vi "Format Metadata.vi"(0 "Tone Cloud in":refnum<class "Tone Cloud.lvclass">, 7 "Prefix":string, 11 "error in (no error)":errorcluster) -> (4 "Tone Cloud out":refnum<class "Tone Cloud.lvclass">, 8 "String":string, 15 "error out":errorcluster)   [LabVIEW 2020, in "Tone Cloud.lvclass"]
uses:
  Tone Cloud.lvclass
  Tone Cloud.lvclass/Tone Cloud.ctl
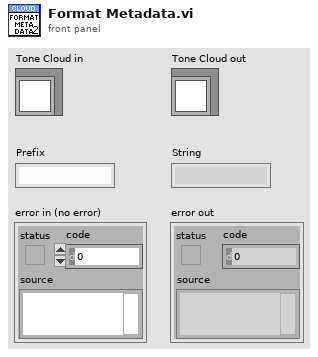
[diagram p1: front panel]
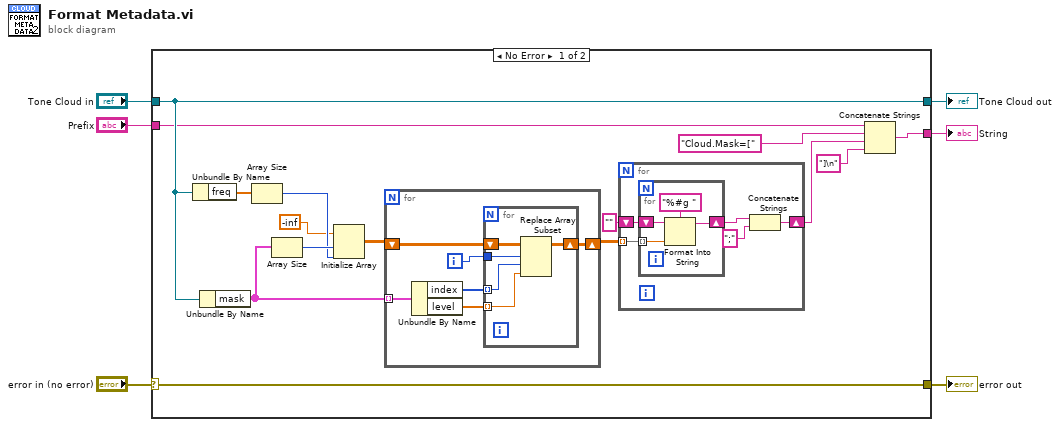
[diagram p0: block diagram]
diagram:
  n1 = case shown="No Error" "error in (no error)" {
    selector: "error in (no error)" -> [w21 w43]
    tunnel: [w21 w43] -> w5
    tunnel: [w20 w42] -> w4
    tunnel: "Tone Cloud in" -> [w20 w42]
    tunnel: "Prefix" -> [w13 _]
    tunnel: [w12 _] -> w1
    frame No Error {
      n2 = Unbundle By Name(w20) -> ("freq"=w19:dbl[])
      n3 = Unbundle By Name(w20) -> ("mask"=w18:cluster{"index":i32[], "level":dbl[]}[])
      n4 = Array Size(array=w19) -> (size(s)=w16:i32)
      n5 = Array Size(array=w18) -> (size(s)=w17:i32)
      n6 = Initialize Array(-inf, w17, w16) -> (w14:dbl[][])
      n7 = for {
        tunnel: w18 -> [w36] mode=indexing
        shift-right: [w31] -> w10
        shift-left: w14 -> [w35]
        i -> [w32]
        n8 = Unbundle By Name(w36) -> ("index"=w33:i32[], "level"=w34:dbl[])
        n9 = for {
          shift-right: [w40] -> w31
          shift-left: w35 -> [w41]
          tunnel: w34 -> [w37] mode=indexing
          tunnel: w33 -> [w38] mode=indexing
          tunnel: w32 -> [w39]
          n10 = Replace Array Subset(array=w41, new element=w37, index (row)=w39, index (col)=w38) -> (w40:dbl[][])
        }
      }
      n11 = for {
        tunnel: w10 -> [w25] mode=indexing
        shift-right: [w22] -> w7
        shift-left: "" -> [w24]
        n12 = for {
          tunnel: w25 -> [w29] mode=indexing
          shift-right: [w27] -> w23
          shift-left: w24 -> [w28]
          n13 = Format Into String(format string="%#g ", initial string=w28, w29) -> (resulting string=w27:string)  [unwired: 1 in, 1 out]
        }
        n14 = Concatenate Strings(w23, ";") -> (w22:string)
      }
      n15 = Concatenate Strings(w13, "Cloud.Mask=[" ("string"), w7, "]\n") -> (w12:string)
    }
    frame Error {
    }
  }
  "error out" <- w5
  "Tone Cloud out" <- w4
  "String" <- w1
